vi "Data Receiver.vi"() -> ()   [LabVIEW 2018]
doc: "Demonstrates how to open a connection to a specified host and port, read the data being sent to the port, and display the data on a chart. This VI is designed to stop if the TCP connection is terminated.\n\n<B>Note:</B> Requires the Simple Data Server.vi located in the same library as this VI."
panel:
  out "Time":string
  out "Bytes to read (dec)":i32
  out "Bytes to read (hex)":string
  out "Complete String after 'Bytes to read'":string
  out "Peak Powers":string[][](array[string])
  out "Peak Wavelengths":string[][](array[string])
  out "System Status":string[][](array[string])
  out "Qty of FBG's":string[](array[string])
  out "OpticalLineNumber":string[](array[string])
  out "Date":string
  out "LineNumber":string
  out "Qty of Optical Lines":string
  in  "Start":bool
  in  "stop":bool
  in  "Address":string="127.0.0.1"
  in  "Port":u16=2055 min=1025 step=1
  # "Instructions:\n1. Adjust the IP address and Port.\n2. Press START."
  # "Separated data"
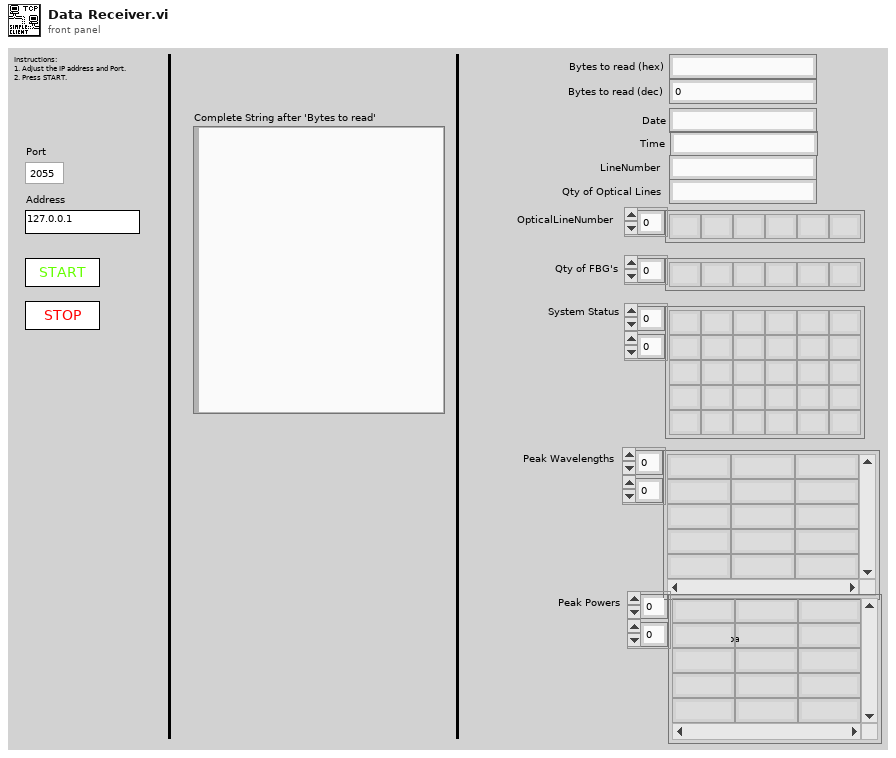
[diagram p1: front panel]
types:
  T1 = enum16{"open", "replace", "create", "open or create", "replace or create", "replace or create with confirmation"}
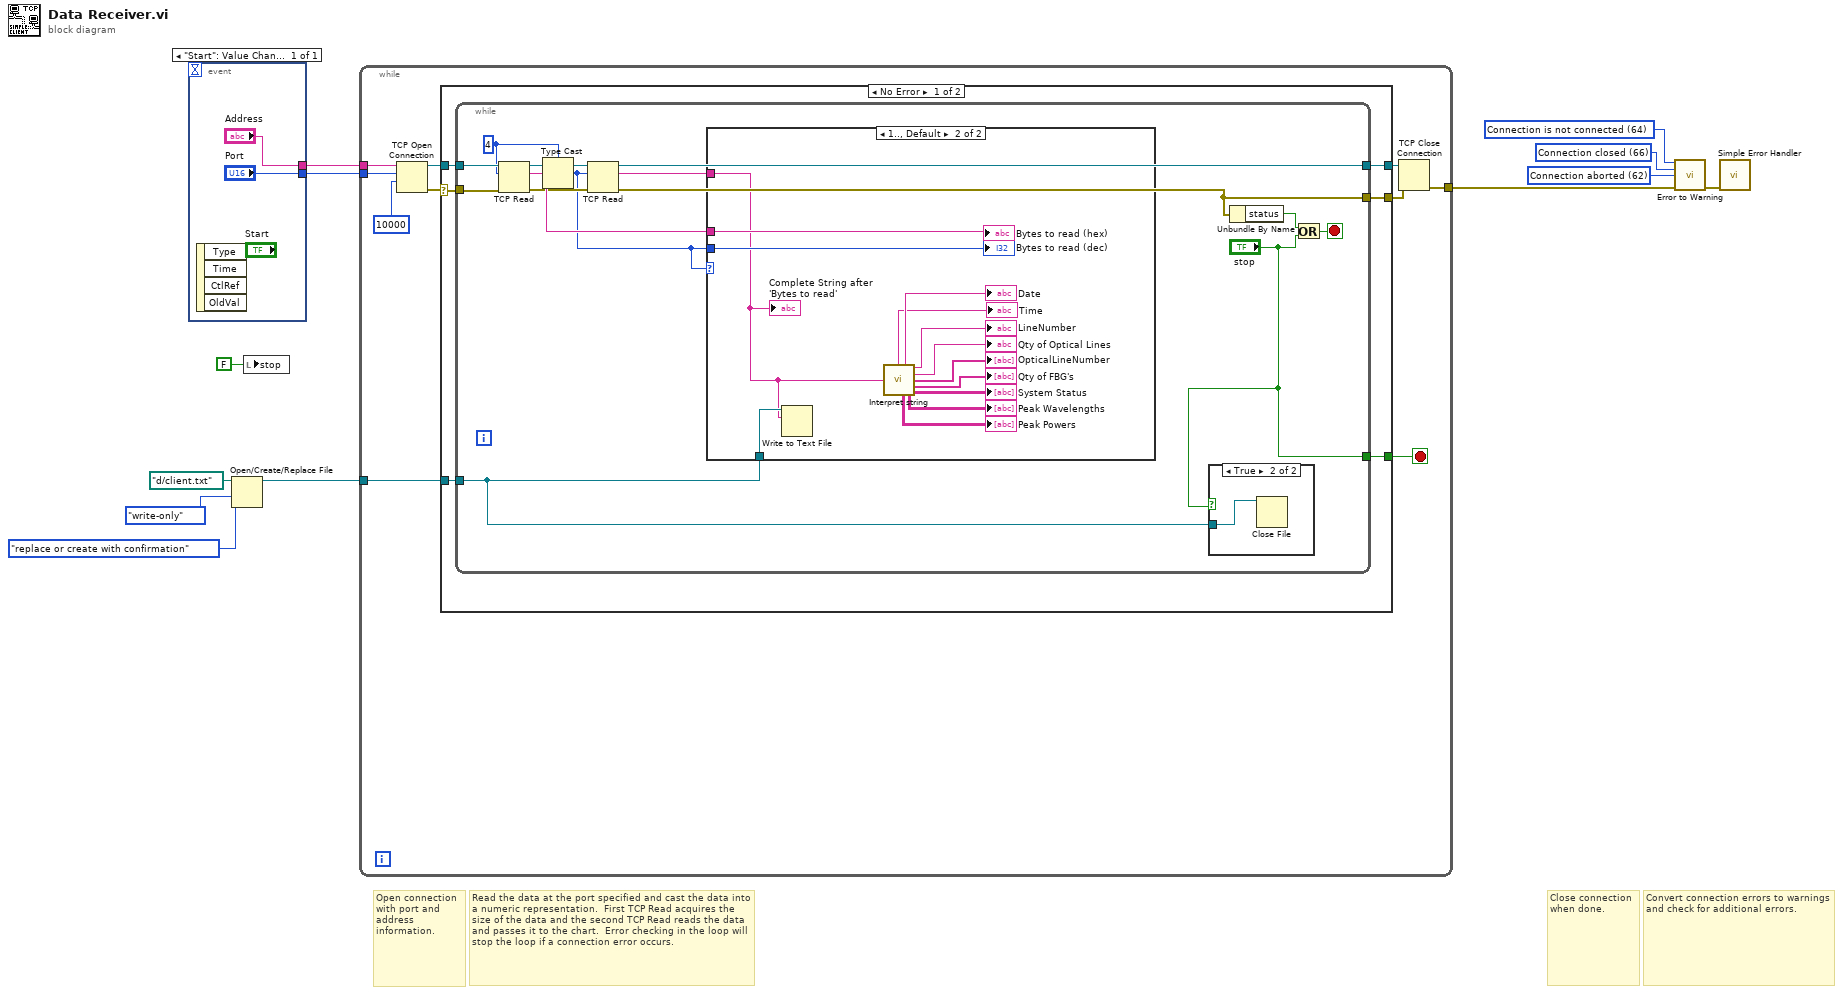
[diagram p0: block diagram]
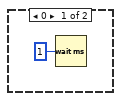
[diagram p3: hidden frame]
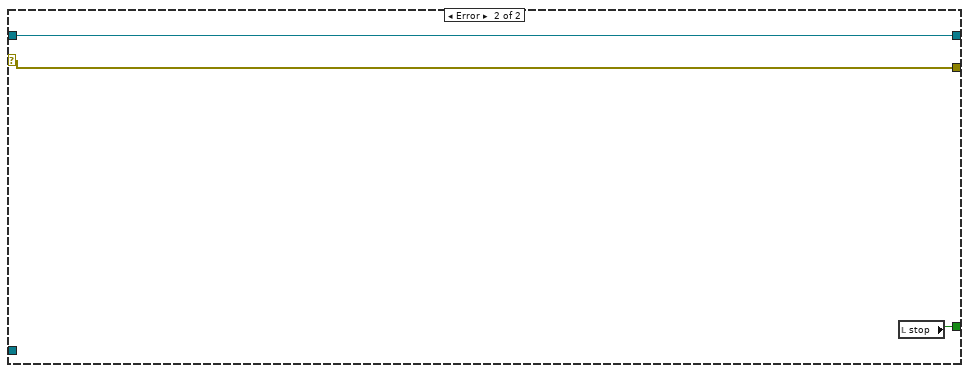
[diagram p4: hidden frame]
diagram:
  w8 = 62 items=["No Error", "Argument Error", "Memory Full", "Out of Zone", "End of File", "File Already Open", "Generic File IO Error", "File Not Found", "File Permission Error", "Disk Full", "Duplicate Path", "Too Many Files Open", "Not Enabled", "Resource File Not Found", "Cannot Add Resource", "Resource Not Found", "Image Not Found", "Image Memory Error", "Pen Does Not Exist", "Config Bad Type", "Config Token Not Found", "Config Parse Error", "Config Memory Error", "Bad External Code Format", "Bad External Code Offset", "External Code Not Present", "Null Window", "Destroy Window Mixup", "Null Menu", "Print Aborted", "Bad Print Record", "Print Driver Error", "Windows Error During Print", "Memory Error During Print", "Print Dialog Error", "Generic Print Error", "Invalid Device Refnum", "Device Not Found", "Device Parameter Error", "Device Unit Error", "Can't Open Device", "Device Call Aborted", "Generic Error", "Cancelled By User", "Object ID Too Low", "Object ID Too High", "Object Not In Heap", "Unknown Heap", "Bad DefProc ID", "DefProc Not In Table", "Message Out Of Range", "Null Method", "Unknown Message", "Manager Call Not Supported", "Bad address", "Connection In progress", "Connection timed out", "Connection is already in progress", "Network attribute not supported", "Network error", "Address in use", "System out of memory", "Connection aborted", "Connection refused", "Connection is not connected", "Connection is already connected", "Connection closed", "Initialize error (interapplication manager)", "Bad occurrence", "Wait on unbound occurrence handler", "Occurrence queue overflow", "Bad path", "Semaphore not signaled", "Unrecognized type (interapplication manager)"] ("1st Error to Convert")
  w9 = 66 items=["No Error", "Argument Error", "Memory Full", "Out of Zone", "End of File", "File Already Open", "Generic File IO Error", "File Not Found", "File Permission Error", "Disk Full", "Duplicate Path", "Too Many Files Open", "Not Enabled", "Resource File Not Found", "Cannot Add Resource", "Resource Not Found", "Image Not Found", "Image Memory Error", "Pen Does Not Exist", "Config Bad Type", "Config Token Not Found", "Config Parse Error", "Config Memory Error", "Bad External Code Format", "Bad External Code Offset", "External Code Not Present", "Null Window", "Destroy Window Mixup", "Null Menu", "Print Aborted", "Bad Print Record", "Print Driver Error", "Windows Error During Print", "Memory Error During Print", "Print Dialog Error", "Generic Print Error", "Invalid Device Refnum", "Device Not Found", "Device Parameter Error", "Device Unit Error", "Can't Open Device", "Device Call Aborted", "Generic Error", "Cancelled By User", "Object ID Too Low", "Object ID Too High", "Object Not In Heap", "Unknown Heap", "Bad DefProc ID", "DefProc Not In Table", "Message Out Of Range", "Null Method", "Unknown Message", "Manager Call Not Supported", "Bad address", "Connection In progress", "Connection timed out", "Connection is already in progress", "Network attribute not supported", "Network error", "Address in use", "System out of memory", "Connection aborted", "Connection refused", "Connection is not connected", "Connection is already connected", "Connection closed", "Initialize error (interapplication manager)", "Bad occurrence", "Wait on unbound occurrence handler", "Occurrence queue overflow", "Bad path", "Semaphore not signaled", "Unrecognized type (interapplication manager)"] ("1st Error to Convert")
  w10 = 64 items=["No Error", "Argument Error", "Memory Full", "Out of Zone", "End of File", "File Already Open", "Generic File IO Error", "File Not Found", "File Permission Error", "Disk Full", "Duplicate Path", "Too Many Files Open", "Not Enabled", "Resource File Not Found", "Cannot Add Resource", "Resource Not Found", "Image Not Found", "Image Memory Error", "Pen Does Not Exist", "Config Bad Type", "Config Token Not Found", "Config Parse Error", "Config Memory Error", "Bad External Code Format", "Bad External Code Offset", "External Code Not Present", "Null Window", "Destroy Window Mixup", "Null Menu", "Print Aborted", "Bad Print Record", "Print Driver Error", "Windows Error During Print", "Memory Error During Print", "Print Dialog Error", "Generic Print Error", "Invalid Device Refnum", "Device Not Found", "Device Parameter Error", "Device Unit Error", "Can't Open Device", "Device Call Aborted", "Generic Error", "Cancelled By User", "Object ID Too Low", "Object ID Too High", "Object Not In Heap", "Unknown Heap", "Bad DefProc ID", "DefProc Not In Table", "Message Out Of Range", "Null Method", "Unknown Message", "Manager Call Not Supported", "Bad address", "Connection In progress", "Connection timed out", "Connection is already in progress", "Network attribute not supported", "Network error", "Address in use", "System out of memory", "Connection aborted", "Connection refused", "Connection is not connected", "Connection is already connected", "Connection closed", "Initialize error (interapplication manager)", "Bad occurrence", "Wait on unbound occurrence handler", "Occurrence queue overflow", "Bad path", "Semaphore not signaled", "Unrecognized type (interapplication manager)"] ("1st Error to Convert")
  # "Convert connection errors to warnings and check for additional errors."
  # "Close connection when done."
  # "Read the data at the port specified and cast the data into a numeric representation.  First TCP Read acquires the size of the data and the second TCP Read reads the data and passes it to the chart.  Error checking in the loop will stop the loop if a connection error occurs."
  # "Open connection\nwith port and \naddress information."
  n1 = event shown="[0] \"Start\": Value Change" {
    selector: _ -> [_]
    dyn-events: _ -> [_]
    timeout: _ -> [_]
    tunnel: ["Address"] -> w7
    tunnel: ["Port"] -> w6
    event "Start": Value Change {
      n2 = event-data() -> ()  [unwired: 1 in, 4 out]
    }
  }
  n3 = Open/Create/Replace File(file path (use dialog)=path "d:/client.txt", operation (0:open)=T1."replace or create with confirmation", access (0:read/write)=enum16{"read/write", "read-only", "write-only"}."write-only") -> (refnum out=w1:refnum<file>)  [unwired: 3 in, 2 out]
  n4 = local write "stop"(FALSE ("stop")) -> ()
  n5 = while {
    tunnel: [w21] -> w12
    tunnel: w7 -> [w20]
    tunnel: w6 -> [w19]
    tunnel: w1 -> [w16]
    stop <- w18 stop-if-true
    n6 = TCP Open Connection(address=w20, remote port or service name=w19, timeout ms (60000)=10000) -> (connection ID=w22:refnum<k5>, error out=w17:errorcluster)  [unwired: 2 in]
    n7 = case shown="No Error" w17 {
      selector: w17 -> [w26 w61]
      tunnel: [w30 w61] -> w24
      tunnel: [w29 w62] -> w23
      tunnel: w22 -> [w28 w62]
      tunnel: [w27 w60] -> w18
      tunnel: w16 -> [w25 _]
      frame No Error {
        n8 = while {
          tunnel: w26 -> [w41]
          tunnel: w28 -> [w42]
          tunnel: [w43] -> w29
          tunnel: [w40] -> w30
          tunnel: ["stop"] -> w27
          tunnel: w25 -> [w33]
          stop <- w38 stop-if-true
          w32 = 4
          n9 = TCP Read(connection ID=w42, bytes to read=w32, error in (no error)=w41) -> (connection ID out=w44:refnum<k5>, data out=w37:string, error out=w35:errorcluster)  [unwired: 2 in]
          n10 = Type Cast(type=w32, x=w37) -> (*(type *) &x=w31:i32)
          n11 = TCP Read(connection ID=w44, bytes to read=w31, error in (no error)=w35) -> (connection ID out=w43:refnum<k5>, data out=w36:string, error out=w40:errorcluster)  [unwired: 2 in]
          n12 = case shown="1.., Default" w31 {
            tunnel: w37 -> [_ w59]
            tunnel: w36 -> [_ w56]
            tunnel: w31 -> [_ w58]
            tunnel: w33 -> [_ w57]
            frame 0 {
              n13 = Wait (ms)(milliseconds to wait=u32 1) -> ()  [unwired: 1 out]
            }
            frame 1.., Default {
              n14 = Write to Text File(file (use dialog)=w57, text=w56) -> ()  [unwired: 2 in, 3 out]
              n15 = call "Interpret string.vi"("Spreadsheet string"=w56) -> ("Time"=→"Time":string, "Date"=→"Date":string, "LineNumber"=→"LineNumber":string, "Qty of Optical Lines"=→"Qty of Optical Lines":string, "OpticalLineNumber"=→"OpticalLineNumber":string[], "Qty of FBG's"=→"Qty of FBG's":string[], "Peak Powers"=→"Peak Powers":string[][], "Peak Wavelengths"=→"Peak Wavelengths":string[][], "System Status"=→"System Status":string[][])  [unwired: 6 in]
              "Complete String after 'Bytes to read'" <- w56
              "Bytes to read (hex)" <- w59
              "Bytes to read (dec)" <- w58
            }
          }
          n16 = case shown="True" "stop" {
            tunnel: w33 -> [_ w45]
            frame False {
            }
            frame True {
              n17 = Close File(refnum=w45) -> ()  [unwired: 1 in, 2 out]
            }
          }
          n18 = Unbundle By Name(w40) -> ("status"=w39:bool)
          n19 = Or(x=w39, y="stop") -> (x .or. y?=w38:bool)
        }
      }
      frame Error {
        n20 = local read "stop"() -> (w60:bool)
      }
    }
    n21 = TCP Close Connection(connection ID=w23, error in (no error)=w24) -> (error out=w21:errorcluster)  [unwired: 1 in, 1 out]
  }
  n22 = call <vilib>:"Error to Warning.vi"("1st Error to Convert"=w10, "2nd Error to Convert"=w9, "3rd Error to Convert"=w8, "error in"=w12) -> ("warning out"=w11:errorcluster)  [unwired: 11 in]
  n23 = call <vilib>:"Simple Error Handler.vi"("error in (no error)"=w11) -> ()  [unwired: 4 in, 5 out]
